vi "Escape Term Name Characters.vi"(11 "terminal name in":string) -> (3 "terminal name out":string)   [LabVIEW 2020, in "Web Service Description.lvlib"]
uses:
  <vilib>/AppBuilder/Engine/WebServiceDescription/Web Service Description.lvlib
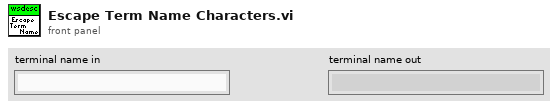
[diagram p1: front panel]
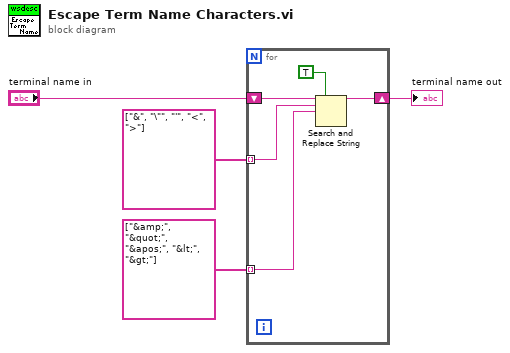
[diagram p0: block diagram]
diagram:
  n1 = for {
    shift-right: [w8] -> w3
    shift-left: "terminal name in" -> [w9]
    tunnel: string[] ["&", "\"", "'", "<", ">"] -> [w6] mode=indexing
    tunnel: string[] ["&amp;", "&quot;", "&apos;", "&lt;", "&gt;"] -> [w5] mode=indexing
    n2 = Search and Replace String(replace all?=TRUE ("replace all? (F)"), input string=w9, search string=w6, replace string=w5) -> (result string=w8:string)  [unwired: 4 in, 3 out]
  }
  "terminal name out" <- w3
